vi "Locate Object.vi"(7 "Tolerance":cluster{"x":dbl, "y":dbl, "a":dbl}={"x"=2.0, "y"=2.0, "a"=2.0}, 8 "error in":errorcluster, 9 "Type":T1, 11 "Object":string="Grippee") -> (0 "error out":errorcluster, 1 "Found":bool, 2 "Range":dbl, 3 "result":cluster{"x":dbl, "y":dbl, "a":dbl}, 4 "Close":bool, 5 "picture":picture)   [LabVIEW 2013]
uses:
  Teach Locations.ctl
  ROS/Code/SubVIs/BaxterCamera.ctl
  ROS/Code/SubVIs/BaxterSide.ctl
  Arm Globals.vi
  <vilib>/Utility/config.llb/Read Key (String).vi
  <vilib>/Utility/config.llb/NI_LVConfig.lvlib
  <vilib>/Analysis/NI_AALBase.lvlib
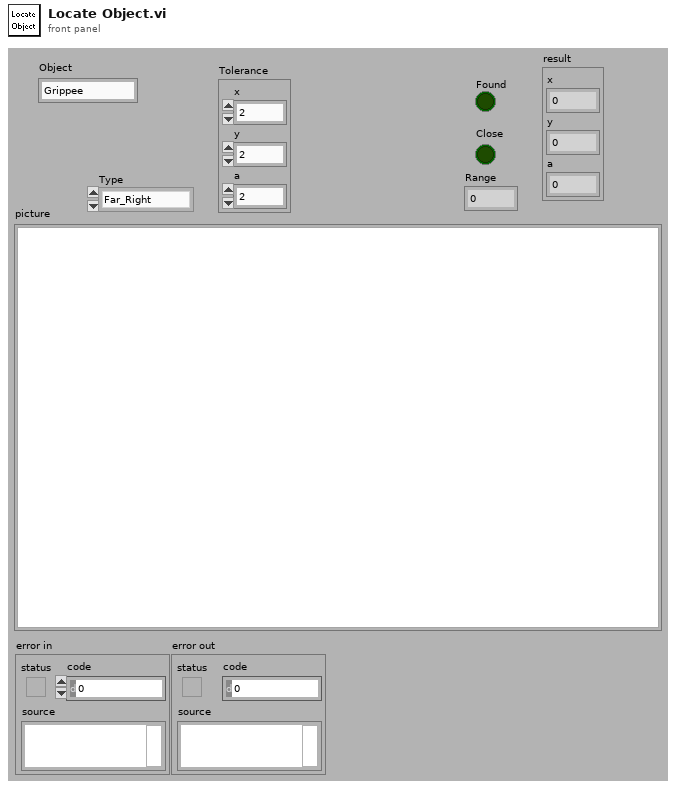
[diagram p1: front panel]
types:
  T1 = typedef "Teach Locations.ctl" = enum16{"Far_Right", "Near_Right", "Far_Left", "Near_Left", "Bottom", "Top", "Right", "Left"}
  T2 = typedef "NI_LVConfig.lvlib/Config Data RefNum.ctl" = refnum<k1>
  T3 = typedef "BaxterSide.ctl" = enum16{"left", "right"}
  T4 = typedef "BaxterCamera.ctl" = enum16{"left_hand_camera", "right_hand_camera", "head_camera"}
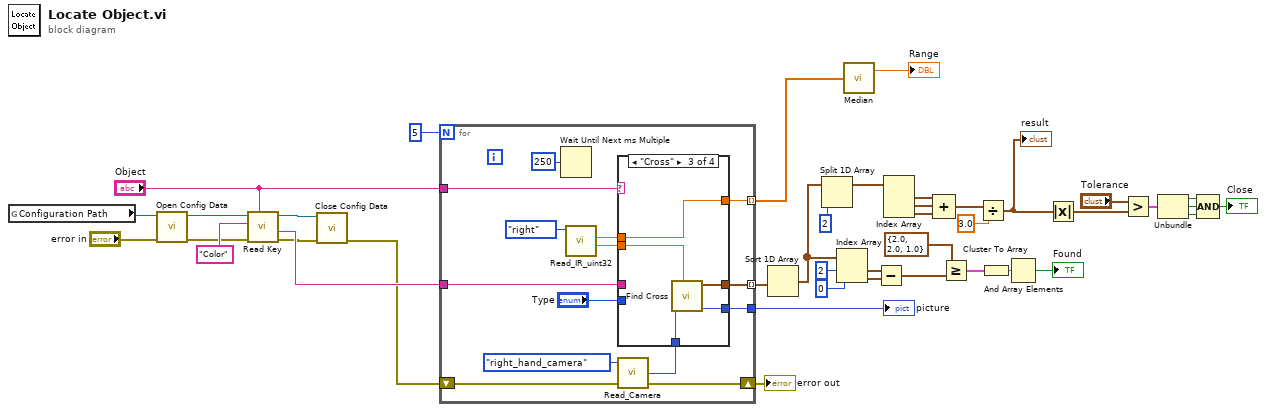
[diagram p0: block diagram]
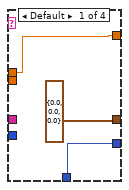
[diagram p2: hidden frame]
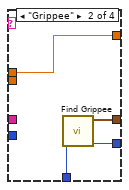
[diagram p3: hidden frame]
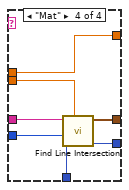
[diagram p4: hidden frame]
diagram:
  n1 = global read "Arm Globals.vi" "Configuration Path"() -> (w8:path)
  n2 = call <vilib>:"Open Config Data.vi"("error in (no error)"="error in", "configuration file path"=w8) -> ("error out"=w1:errorcluster, "refnum"=w5:T2)  [unwired: 7 in, 1 out]
  n3 = call-poly <vilib>:"Read Key.vi"("section"="Object", "error in (no error)"=w1, "key"="Color", "refnum"=w5) -> ("error out"=w3:errorcluster, "value"=w9:string, "refnum out"=w4:T2)  [unwired: 4 in, 1 out]
  n4 = call <vilib>:"Close Config Data.vi"("error in (no error)"=w3, "refnum"=w4) -> ("error out"=w2:errorcluster)  [unwired: 8 in, 1 out]
  n5 = for {
    N: 5 -> [_]
    tunnel: [w54] -> w41
    shift-right: [w50] -> w40
    shift-left: w2 -> [w51]
    tunnel: [w49] -> w38 mode=indexing
    tunnel: [w46] -> w12 mode=indexing
    tunnel: "Object" -> [w44]
    tunnel: w9 -> [w43]
    n6 = Wait Until Next ms Multiple(millisecond multiple=u32 250) -> ()  [unwired: 1 out]
    n7 = call "Read_IR_uint32.vi"("Side"=BaxterSide."right") -> ("mm/pixel"=w47:dbl, "Distance"=w45:dbl)  [unwired: 4 in, 2 out]
    n8 = call "Read_Camera.vi"("Camera"=BaxterCamera."right_hand_camera", "error in"=w51) -> ("picture"=w52:picture, "error out"=w50:errorcluster)  [unwired: 3 in, 1 out]
    n9 = case shown="\"Cross\"" w44 {
      tunnel: [w58 w62 w67 w74] -> w54
      tunnel: w52 -> [w58 w61 w66 w73]
      tunnel: [cluster{"x":dbl, "y":dbl, "a":dbl} {"x"=0.0, "y"=0.0, "a"=0.0} ("Result") w60 w65 w72] -> w49
      tunnel: w47 -> [_ _ w63 w70]
      tunnel: [w56 w59 w64 w71] -> w46
      tunnel: w45 -> [w56 w59 w64 w71]
      tunnel: w43 -> [_ _ _ w69]
      tunnel: "Type" -> [_ _ _ w68]
      frame Default {
      }
      frame "Grippee" {
        n10 = call "Find Grippee.vi"("picture"=w61) -> ("picture"=w62:picture, "result"=w60:cluster{"x":dbl, "y":dbl, "a":dbl})  [unwired: 7 in, 2 out]
      }
      frame "Cross" {
        n11 = call "Find Cross.vi"("mm/pixel"=w63, "picture"=w66) -> ("picture"=w67:picture, "Result"=w65:cluster{"x":dbl, "y":dbl, "a":dbl})  [unwired: 6 in, 2 out]
      }
      frame "Mat" {
        n12 = call "Find Line Intersection.vi"("mm/pixel"=w70, "picture"=w73, "Type"=w68, "Color"=w69) -> ("picture"=w74:picture, "Result"=w72:cluster{"x":dbl, "y":dbl, "a":dbl})  [unwired: 4 in, 2 out]
      }
    }
  }
  "picture" <- w41
  "error out" <- w40
  n13 = Sort 1D Array(array=w38) -> (sorted array=w30:cluster{"x":dbl, "y":dbl, "a":dbl}[])
  n14 = Split 1D Array(array=w30, index=2) -> (first subarray=w28:cluster{"x":dbl, "y":dbl, "a":dbl}[])  [unwired: 1 out]
  n15 = Index Array(array=w30, index #1=2 ("index"), index #2=0 ("index")) -> (element #1=w35:cluster{"x":dbl, "y":dbl, "a":dbl}, element #2=w34:cluster{"x":dbl, "y":dbl, "a":dbl})
  n16 = call <vilib>:"Median.vi"("X"=w12) -> ("median"=→"Range":dbl)  [unwired: 1 out]
  n17 = Subtract(x=w35, y=w34) -> (x-y=w33:cluster{"x":dbl, "y":dbl, "a":dbl})
  n18 = Index Array(array=w28) -> (element #1=w27:cluster{"x":dbl, "y":dbl, "a":dbl}, element #2=w26:cluster{"x":dbl, "y":dbl, "a":dbl}, element #3=w25:cluster{"x":dbl, "y":dbl, "a":dbl})  [unwired: 3 in]
  n19 = Compound Arithmetic op=ADD(w27, w26, w25) -> (w24:cluster{"x":dbl, "y":dbl, "a":dbl})
  n20 = Greater Or Equal?(x=cluster{"x":dbl, "y":dbl, "a":dbl} {"x"=2.0, "y"=2.0, "a"=1.0}, y=w33) -> (x >= y?=w32:cluster{"x":bool, "y":bool, "a":bool})
  n21 = Divide(x=w24, y=3.0) -> (x/y=w15:cluster{"x":dbl, "y":dbl, "a":dbl})
  "result" <- w15
  n22 = Cluster To Array(cluster=w32) -> (array=w31:bool[])
  n23 = And Array Elements(Boolean array=w31) -> (logical AND=→"Found":bool)
  n24 = Absolute Value(x=w15) -> (abs(x)=w17:cluster{"x":dbl, "y":dbl, "a":dbl})
  n25 = Greater?(x="Tolerance", y=w17) -> (0:w21:cluster{"x":bool, "y":bool, "a":bool})
  n26 = Unbundle(w21) -> ("x"=w20:bool, "y"=w19:bool, "a"=w18:bool)
  n27 = Compound Arithmetic op=AND(w20, w19, w18) -> (→"Close":bool)
